vi "Limelight Set Mode Vision Processor.vi"(11 "Vision Processor":bool) -> ()   [LabVIEW 2020]
uses:
  <vilib>/Rock Robotics/Network Tables/NT Write Number.vi
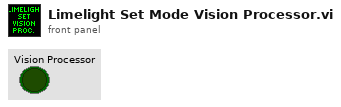
[diagram p1: front panel]
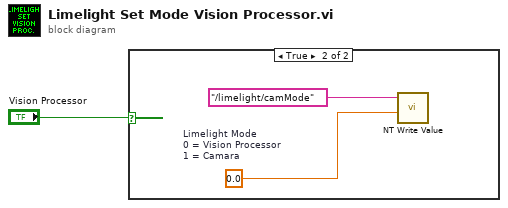
[diagram p0: block diagram]
diagram:
  n1 = case shown="True" "Vision Processor" {
    frame False {
    }
    frame True {
      w2 = 0.0  # Limelight Mode 0 = Vision Processor 1 = Camara
      n2 = call-poly <vilib>:"NT Write Value.vi"("Numeric"=w2, "Name"="/limelight/camMode") -> ()  [unwired: 9 in, 1 out]
    }
  }
